vi "load_class.vi"(8 "error in (no error)":errorcluster, 11 "class":path) -> (0 "error out":errorcluster, 3 "lv_build_plugin":refnum<class "lv-builder.lvclass">)   [LabVIEW 2015, in "lv-builder.lvlib"]
uses:
  lv-builder.lvlib
  class/lv-builder.lvclass
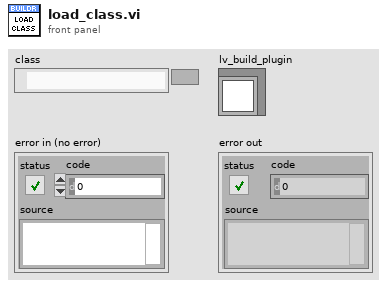
[diagram p1: front panel]
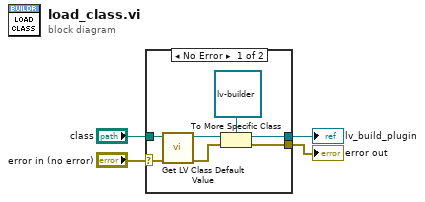
[diagram p0: block diagram]
diagram:
  n1 = case shown="No Error" "error in (no error)" {
    selector: "error in (no error)" -> [w6 w12]
    tunnel: [w9 _] -> w4
    tunnel: [w8 w12] -> w3
    tunnel: "class" -> [w7 _]
    frame No Error {
      n2 = call <vilib>:"Get LV Class Default Value.vi"("error in (no error)"=w6, "class path"=w7) -> ("error out"=w10:errorcluster, "object"=w11:refnum<class>)  [unwired: 8 in]
      n3 = To More Specific Class(target class=refnum<class "lv-builder.lvclass"> refnum ("lv-build.lvlib:lv-build.lvclass"), reference=w11, error in=w10) -> (specific class reference=w9:refnum<class "lv-builder.lvclass">, error out=w8:errorcluster)
    }
    frame Error {
    }
  }
  "error out" <- w3
  "lv_build_plugin" <- w4
